vi "IV_DCM.vi"(4 "2812 -A Params In":T10={"Auto Range?"=FALSE, "Man / Selected\nRange"=enum."10V", "Enable Digital\nFilter?"=TRUE, "Filter Type"=enum."Moving", "Filter Count"=10, "Filter\nWindow (%)"=0.01, "Enable Analog\nFilter?"=FALSE, "NPLCs"=2} {"Filter\nWindow (%)" min=0.0 max=10.0 step=0.01 format="%.2f"; "Filter Count" min=1 max=100; "NPLCs" min=1 max=10}, 6 "Differential Cond Params In":T1={"Start Value (A)"=0.0, "Stop Value (A)"=1e-05, "Step Size (A)"=1e-06, "Delta Value (A)"=1e-06, "Delay (s)"=0.002, "Abort On\nCompliance?"=FALSE} {"Delay (s)" min=0.001 max=9999.999 format="%.3f"; "Delta Value (A)" min=0.0 max=0.105 format="%.3p"; "Step Size (A)" min=0.0 max=0.105 format="%.3p"; "Stop Value (A)" min=-0.105 max=0.105 format="%.3p"; "Start Value (A)" min=-0.105 max=0.105 format="%.3p"}, 8 "error in (no error)":errorcluster, 11 "Resource In":refnum<visa-resource-name>) -> (0 "error out":errorcluster, 1 "Voltage (V)":sgl[](array[numeric]), 2 "Current (A)":sgl[](array[numeric]), 3 "Resource Out (dupl)":refnum<visa-resource-name>)   [LabVIEW 2024]
doc: "This VI does I-V measurement using differential conductance mode. The output is arrays of current and voltages."
uses:
  <instrlib>/Keithley 622x LV 2009/Configure/2182 -A/Low Level/Typedefs/KE2182 -- Voltage Ranges.ctl
  <instrlib>/Keithley 622x LV 2009/Configure/2182 -A/Low Level/Typedefs/KE2182 -- Filter Type.ctl
  <instrlib>/Keithley 622x LV 2009/Configure/2182 -A/Low Level/Typedefs/KE2182 -- Filter Count.ctl
  <instrlib>/Keithley 622x LV 2009/Configure/2182 -A/Low Level/Typedefs/KE2182 -- Filter Window.ctl
  <instrlib>/Keithley 622x LV 2009/Configure/2182 -A/Low Level/Typedefs/KE2182 -- NPLCs.ctl
  <instrlib>/Keithley 622x LV 2009/Configure/Delta PDelta DCon Modes/Typedefs/KE622x -- DCon Mode Params.ctl
  <instrlib>/Keithley 622x LV 2009/Configure/Delta PDelta DCon Modes/Low Level/Typedefs/KE622x -- DCon Mode Start Stop Level.ctl
  <instrlib>/Keithley 622x LV 2009/Configure/Delta PDelta DCon Modes/Low Level/Typedefs/KE622x -- DCon Mode Step Delta Size.ctl
  <instrlib>/Keithley 622x LV 2009/Configure/Delta PDelta DCon Modes/Low Level/Typedefs/KE622x -- Delta DCon Mode Delay.ctl
  <instrlib>/Keithley 622x LV 2009/Configure/Units/Typedefs/KE622x -- Voltage Meas Units.ctl
  <instrlib>/Keithley 622x LV 2009/Configure/Format/Typedefs/KE622x -- Optional Meas Elements.ctl
  <instrlib>/Keithley 622x LV 2009/Keithley 622x.lvlib
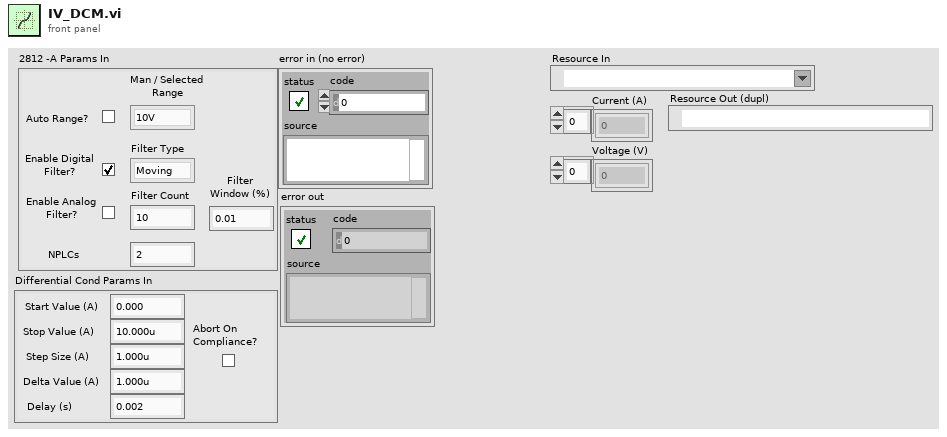
[diagram p1: front panel]
types:
  T1 = typedef "Keithley 622x.lvlib/KE622x -- DCon Mode Params.ctl" = cluster{"Start Value (A)":T2, "Stop Value (A)":T2, "Step Size (A)":T3, "Delta Value (A)":T3, "Delay (s)":T4, "Abort On\nCompliance?":bool}
  T2 = typedef "Keithley 622x.lvlib/KE622x -- DCon Mode Start Stop Level.ctl" = dbl
  T3 = typedef "Keithley 622x.lvlib/KE622x -- DCon Mode Step Delta Size.ctl" = dbl
  T4 = typedef "Keithley 622x.lvlib/KE622x -- Delta DCon Mode Delay.ctl" = dbl
  T5 = typedef "Keithley 622x.lvlib/KE2182 -- Voltage Ranges.ctl" = enum16{"10mV", "100mV", "1V", "10V", "100V"}
  T6 = typedef "Keithley 622x.lvlib/KE2182 -- Filter Type.ctl" = enum16{"Moving", "Repeat"}
  T7 = typedef "Keithley 622x.lvlib/KE2182 -- Filter Count.ctl" = u32
  T8 = typedef "Keithley 622x.lvlib/KE2182 -- Filter Window.ctl" = dbl
  T9 = typedef "Keithley 622x.lvlib/KE2182 -- NPLCs.ctl" = u32
  T10 = cluster{"Auto Range?":bool, "Man / Selected\nRange":T5, "Enable Digital\nFilter?":bool, "Filter Type":T6, "Filter Count":T7, "Filter\nWindow (%)":T8, "Enable Analog\nFilter?":bool, "NPLCs":T9}
  T11 = typedef "Keithley 622x.lvlib/KE622x -- Optional Meas Elements.ctl" = cluster{"Timstamp?":bool, "Reading Num?":bool, "Source Value?":bool, "Compliance?":bool, "Average Voltage?":bool}
  T12 = typedef "Keithley 622x.lvlib/KE622x -- Voltage Meas Units.ctl" = enum16{"Volts", "Ohms", "Watts", "Siemens"}
  T13 = typedef "Keithley 622x.lvlib/KE622x -- Trace Buf.ctl" = cluster{"Additional Valid Arrays":T11, "Reading Num":u32[], "Timestamp (secs)":sgl[], "Source Val (A)":sgl[], "Reading":sgl[], "Average Voltage (V)":sgl[], "Compliance?":bool[]}
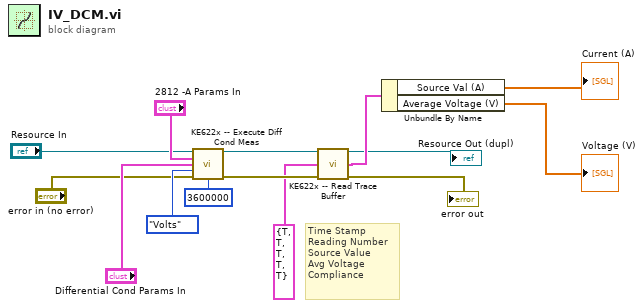
[diagram p0: block diagram]
diagram:
  # "Time Stamp\nReading Number\nSource Value\nAvg Voltage\nCompliance"
  n1 = call <instrlib>:"KE622x -- Execute Diff Cond Meas.vi"("Resource In"="Resource In", "2812 -A Params In"="2812 -A Params In", "Differential Cond Params In"="Differential Cond Params In", "Meas Units"=KE622x_--_Voltage_Meas_Units."Volts", "error in (no error)"="error in (no error)", "Timeout (20000 ms)"=u32 3600000) -> ("Resource Out (dupl)"=w14:refnum<visa-resource-name>, "error out"=w13:errorcluster)  [unwired: 4 in, 4 out]
  n2 = call <instrlib>:"KE622x -- Read Trace Buffer.vi"("Resource In"=w14, "Meas Elements To Return"=T11 {"Timstamp?"=TRUE, "Reading Num?"=TRUE, "Source Value?"=TRUE, "Compliance?"=TRUE, "Average Voltage?"=TRUE}, "error in (no error)"=w13) -> ("Resource Out (dupl)"=→"Resource Out (dupl)":refnum<visa-resource-name>, "Trace Buf"=w9:T13, "error out"=→"error out":errorcluster)  [unwired: 10 in]
  n3 = Unbundle By Name(w9) -> ("Source Val (A)"=→"Current (A)":sgl[], "Average Voltage (V)"=→"Voltage (V)":sgl[])
